vi "GSI-HVSwitch2.close interface.vi"(0 "i ref in":refnum<vi>, 3 "ms timeout (10000)":i32=10000, 5 "error in (no error)":errorcluster) -> (14 "i ref out":refnum<vi>, 17 "timed out":bool, 19 "error out":errorcluster)   [LabVIEW 2014, in "GSI-HVSwitch2.lvlib"]
doc: "Closes the interface to the instrument. This method must be called after communicating with the instrument.\n\nLicense Agreement for this software:\n\nCopyright (C)\nGesellschaft für Schwerionenforschung, GSI\nPlanckstr. 1\n64291 Darmstadt\nGermany\n\nContact: D.Beck@gsi.de \n\nThis program is free software; you can redistribute it and/or modify it under the terms of the GNU General Public License as published by the Free Software Foundation; either version 2 of the license, or (at your option) any later version.\n\nThis program is distributed in the hope that it will be useful, but WITHOUT ANY WARRANTY; without even the implied warranty of MERCHANTABILITY or FITNESS FOR A PARTICULAR PURPOSE. See the GNU General License for more details (http://www.gnu.org).\n\nGesellschaft für Schwerionenforschung, GSI\nPlanckstr. 1, 64291 Darmstadt, Germany\nFor all questions and ideas contact: M.Richter@gsi.de, H.Brand@gsi.de or D.Beck@gsi.de.\nLast update: 17-JUN-2004"
uses:
  GSI-HVSwitch2.lvlib
  CSCore/CSApplicationBaseClasses/DeviceBase/DeviceBase.lvlib
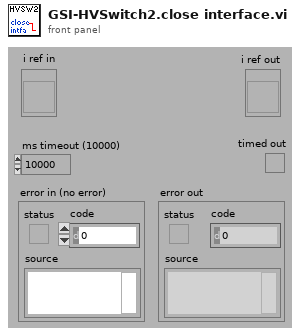
[diagram p1: front panel]
types:
  T1 = typedef "GSI-HVSwitch2.lvlib/GSI-HVSwitch2.i attribute.ctl" = cluster{"SDEX VISA Cluster":T2, "SetVoltage SW0":dbl, "SetVoltage SW1":dbl, "ActTempAmp":dbl, "ActTempPS1":dbl, "ActTempPS2":dbl, "mode":T5, "interfaceInitialized":bool, "serviceIDs":cluster{"nomVoltage0ID":i32, "nomVoltage1ID":i32, "actTempAmpID":i32, "actTempPS1ID":i32, "actTempPS2ID":i32, "modeID":i32}, "usedChannels":i32}
  T2 = typedef "SDEXDriver.lvlib/SDEX.VISA Control.ctl" = cluster{"VISA resource name":refnum<visa-resource-name>, "HEX address":u16, "VISA Timeout Value (1000 ms)":u32, "Lock Timeout (1000 ms)":u32, "semaphore":T3, "Baud rate":u32, "revision":T4, "deviceInfo":string}
  T3 = typedef "Semaphore RefNum" = refnum<k1>
  T4 = typedef "SDEXDriver.lvlib/SDEX.revisionType.ctl" = enum16{"unknown", "hvamp3", "hvswi1", "htrp0", "WDG0"}
  T5 = typedef "GSI-HVSwitch2.lvlib/GSI-HVSwitch2.mode.ctl" = enum16{"unknown", "switch", "stepper"}
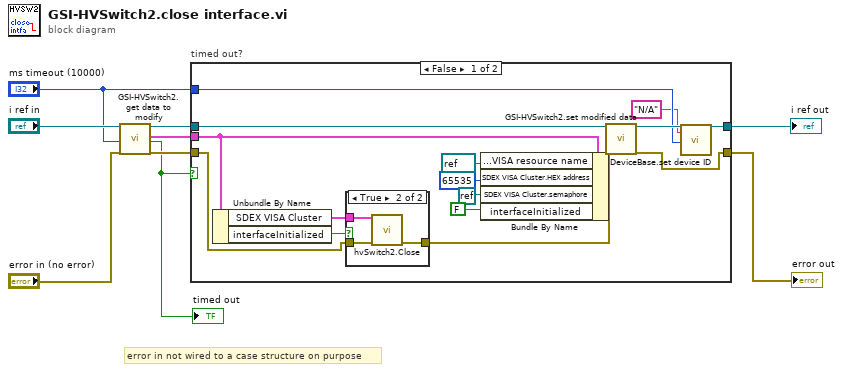
[diagram p0: block diagram]
diagram:
  # "error in not wired to a case structure on purpose"
  n1 = call "GSI-HVSwitch2.get data to modify.vi"("i ref in"="i ref in", "ms timeout (10000)"="ms timeout (10000)", "error in (no error)"="error in (no error)") -> ("i ref out"=w7:refnum<vi>, "i attribute"=w2:T1, "timed out"=w3:bool, "error out"=w5:errorcluster)  [unwired: 13 in]
  "timed out" <- w3
  n2 = case "timed out?" shown="False" w3 {
    tunnel: [w14 w31] -> w6
    tunnel: w7 -> [w21 w31]
    tunnel: [w13 w30] -> w4
    tunnel: w5 -> [w10 w30]
    tunnel: w2 -> [w24 _]
    tunnel: "ms timeout (10000)" -> [w12 _]
    frame False {
      n3 = Unbundle By Name(w24) -> ("SDEX VISA Cluster"=w25:T2, "interfaceInitialized"=w17:bool)
      n4 = case shown="True" w17 {
        tunnel: w25 -> [_ w29]
        tunnel: w10 -> [w26 w28]
        tunnel: [w26 w27] -> w22
        frame False {
        }
        frame True {
          n5 = call "hvSwitch2.Close.vi"("SDEX VISA Cluster"=w29, "error in (no error)"=w28) -> ("error out"=w27:errorcluster)  [unwired: 13 in]
        }
      }
      n6 = Bundle By Name(cluster=w24, "SDEX VISA Cluster.VISA resource name"=refnum<visa-resource-name> refnum, "SDEX VISA Cluster.HEX address"=u16 65535 ("SDEX VISA Cluster.address"), "SDEX VISA Cluster.semaphore"=refnum<k0> refnum ("Not a Refnum Constant"), "interfaceInitialized"=FALSE) -> (w23:T1)
      n7 = call "GSI-HVSwitch2.set modified data.vi"("i ref in"=w21, "i attribute"=w23, "error in (no error)"=w22) -> ("i ref out"=w15:refnum<vi>, "error out"=w13:errorcluster)  [unwired: 15 in]
      n8 = call "DeviceBase.set device ID.vi"("i ref in"=w15, "deviceID"="N/A", "ms timeout (10000)"=w12) -> ("i ref out"=w14:refnum<vi>)  [unwired: 14 in, 2 out]
    }
    frame True {
    }
  }
  "error out" <- w4
  "i ref out" <- w6
